vi "Create.vi"(8 "error in (no error)":errorcluster, 9 "debug mode (F)":bool, 10 "Engine Data Ref":T1 {"Ptr.End" format="%.0x"; "Ptr.Beg" format="%.0x"}, 11 "Device Item Ref":T2=18446744073709551615 format="%.0x") -> (0 "error out":errorcluster, 3 "VeriStand Framework out":refnum<class "VeriStand DSF.Framework.lvclass">)   [LabVIEW 2017, in "Data Sharing Framework Engine.lvlib" / "VeriStand DSF.Framework.lvclass"]
uses:
  VeriStand DSF.Framework.lvclass
  VeriStand Framework Configuration/VeriStand DSF.Framework.Configuration.lvclass
  Data Sharing Framework Engine.lvlib
  Builds/Current/Data Sharing Framework Core/Data Sharing Framework Core.lvlibp/Engine/Internal/Debug/Debug Flags/Debug Flags.lvclass
  Builds/Current/Data Sharing Framework Core/Data Sharing Framework Core.lvlibp/Engine/Internal/Memory/Double Pointer/Double Pointer.lvclass
  Builds/Current/Data Sharing Framework Core/Data Sharing Framework Core.lvlibp/Engine/Internal/Debug/Debug Flags FIFO/Debug Flags FIFO.lvclass
  Builds/Current/Data Sharing Framework Core/Data Sharing Framework Core.lvlibp/Engine/Framework/Framework.lvclass
  C:/github/data-sharing-framework/Data Sharing Framework/Builds/Current/Data Sharing Framework Core/Data Sharing Framework Core.lvlibp/Engine/Framework/Framework.lvclass
  C:/github/data-sharing-framework/Data Sharing Framework/Builds/Current/Data Sharing Framework Core/Data Sharing Framework Core.lvlibp/1abvi3w/vi.lib/National Instruments/Memory Manager/Classes/Pointer/Memory.Pointer.lvclass
  C:/github/data-sharing-framework/Data Sharing Framework/Builds/Current/Data Sharing Framework Core/Data Sharing Framework Core.lvlibp/Engine/Internal/Configuration Classes/Framework Configuration/Framework Configuration.lvclass
  C:/github/data-sharing-framework/Data Sharing Framework/Builds/Current/Data Sharing Framework Core/Data Sharing Framework Core.lvlibp/Engine/Internal/Configuration Classes/Configuration/Configuration.lvclass
  <vilib>/NI Veristand/Custom Device API/Custom Device Item Ref.ctl
  <vilib>/NI VeriStand/Custom Device API/Custom Device API.lvlib
  <vilib>/NI Veristand/Custom Device API/Data Table Ref.ctl
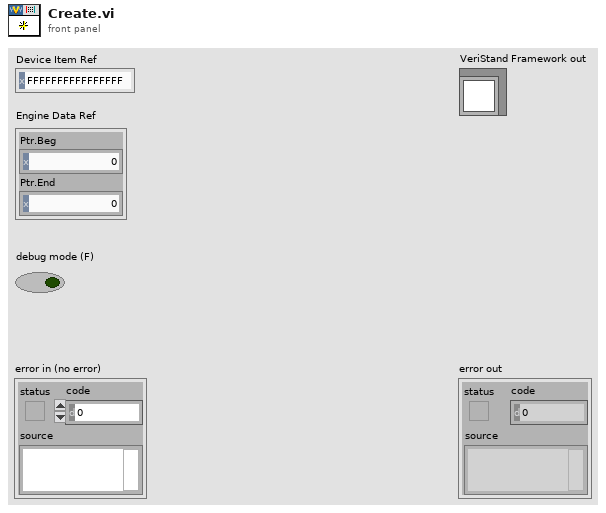
[diagram p1: front panel]
types:
  T1 = typedef "Custom Device API.lvlib/Data Table Ref.ctl" = cluster{"Ptr.Beg":u64, "Ptr.End":u64}
  T2 = typedef "Custom Device API.lvlib/Custom Device Item Ref.ctl" = u64
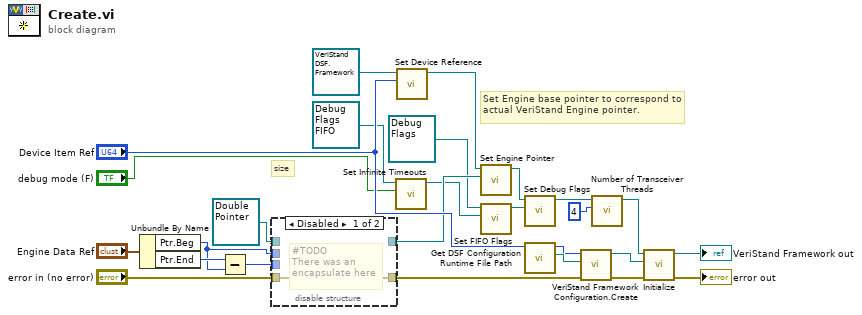
[diagram p0: block diagram]
diagram:
  # "size"
  # "Set Engine base pointer to correspond to actual VeriStand Engine pointer."
  n1 = Unbundle By Name("Engine Data Ref") -> ("Ptr.Beg"=w21:u64, "Ptr.End"=w23:u64)
  n2 = Subtract(x=w23, y=w21) -> (x-y=w22:u64)
  n3 = disable-structure shown="Disabled" {
    disable-tunnel: refnum<class "Double Pointer.lvclass"> refnum ("Engine Channels Pointer") -> [_ w29]
    disable-tunnel: w22 -> [_ _]
    disable-tunnel: w21 -> [_ _]
    disable-tunnel: "error in (no error)" -> [w27 w28]
    disable-tunnel: [w27 w28] -> w13
    disable-tunnel: [_ w29] -> w17
    frame Disabled {
      # "#TODO\nThere was an\nencapsulate here"
    }
    frame Enabled {
    }
  }
  n4 = call "Set Infinite Timeouts.vi"("infinite timeouts"="debug mode (F)", "FIFO Debug Flags in"=refnum<class "Debug Flags FIFO.lvclass"> refnum) -> ("FIFO Debug Flags out"=w12:refnum<class "Debug Flags FIFO.lvclass">)  [unwired: 9 in]
  n5 = call "Set Device Reference.vi"("Device Item Ref"="Device Item Ref", "VeriStand Framework in"=refnum<class "VeriStand DSF.Framework.lvclass"> refnum) -> ("VeriStand Framework out"=w24:refnum<class "VeriStand DSF.Framework.lvclass">)  [unwired: 9 in]
  n6 = call "Set Engine Pointer.vi"("Engine Pointer"=w17, "Framework in"=w24) -> ("Framework out"=w10:refnum<class "VeriStand DSF.Framework.lvclass">)  [unwired: 9 in]
  n7 = call "Set FIFO Flags.vi"("FIFO"=w12, "Debug Flags in"=refnum<class "Debug Flags.lvclass"> refnum) -> ("Debug Flags out"=w8:refnum<class "Debug Flags.lvclass">)  [unwired: 9 in]
  n8 = call "Set Debug Flags.vi"("Debug Flags"=w8, "Framework in"=w10) -> ("Framework out"=w9:refnum<class "VeriStand DSF.Framework.lvclass">)  [unwired: 9 in]
  n9 = call "Get DSF Configuration Runtime File Path.vi"("Item Ref in"="Device Item Ref") -> ("Path"=w15:path, "Item Ref out"=w14:T2)  [unwired: 7 in, 2 out]
  n10 = call "VeriStand Framework Configuration.Create.vi"("error in (no error)"=w13, "configuration path"=w15, "Device Item Ref"=w14) -> ("error out"=w1:errorcluster, "VeriStand Framework Configuration"=w4:refnum<class "VeriStand DSF.Framework.Configuration.lvclass">)  [unwired: 7 in]
  n11 = call "Number of Transceiver Threads.vi"("transceiver count"=4, "Framework in"=w9) -> ("Framework out"=w5:refnum<class "VeriStand DSF.Framework.lvclass">)  [unwired: 8 in, 1 out]
  n12 = call "Initialize.vi"("error in (no error)"=w1, "Framework Configuration"=w4, "Framework type"=w5) -> ("error out"=→"error out":errorcluster, "Framework out"=→"VeriStand Framework out":refnum<class "VeriStand DSF.Framework.lvclass">)  [unwired: 7 in]
